vi "sweep(SubVI).vi"(0 "data":refnum<queue>, 1 "类型":enum16{"temp", "field", "position"}(ring), 2 "Instrument Ref In":refnum<k24>, 4 "config":refnum<queue>, 5 "steps number":i32, 7 "ch str":string, 9 "Field":dbl=300.0, 11 "Mode":i32(ring) items=["Persistent", "Driven"], 13 "Field 2":dbl=300.0, 14 "Rate、speed":dbl=10.0) -> (8 "错误输出":errorcluster)   [LabVIEW 2019, in "SubVI.lvlib"]
uses:
  SubVI.lvlib
  lib/QDInstrument.dll
  config.ctl
panel:
  out "Field\nStatus 3":i32(ring) items=["MagnetUnknown"=0, "StablePersistent"=1, "WarmingSwitch"=2, "CoolingSwitch"=3, "StableDriven"=4, "Iterating"=5, "Charging"=6, "Discharging"=7, "CurrentError"=8, "MagnetFailure"=15]
  out "Temperature\nStatus 2":i32(ring) items=["TemperatureUnknown"=0, "Stable"=1, "Tracking"=2, "Near"=5, "Chasing"=6, "Filling"=7, "Standby"=10, "Disabled"=13, "ImpedanceNotFunction"=14, "TempFailure"=15]
  out "Temperature\nStatus":i32(ring) items=["TemperatureUnknown"=0, "Stable"=1, "Tracking"=2, "Near"=5, "Chasing"=6, "Filling"=7, "Standby"=10, "Disabled"=13, "ImpedanceNotFunction"=14, "TempFailure"=15]
  out "Field\nStatus 2":i32(ring) items=["MagnetUnknown"=0, "StablePersistent"=1, "WarmingSwitch"=2, "CoolingSwitch"=3, "StableDriven"=4, "Iterating"=5, "Charging"=6, "Discharging"=7, "CurrentError"=8, "MagnetFailure"=15]
  # "(真是通道1，假是通道2)"
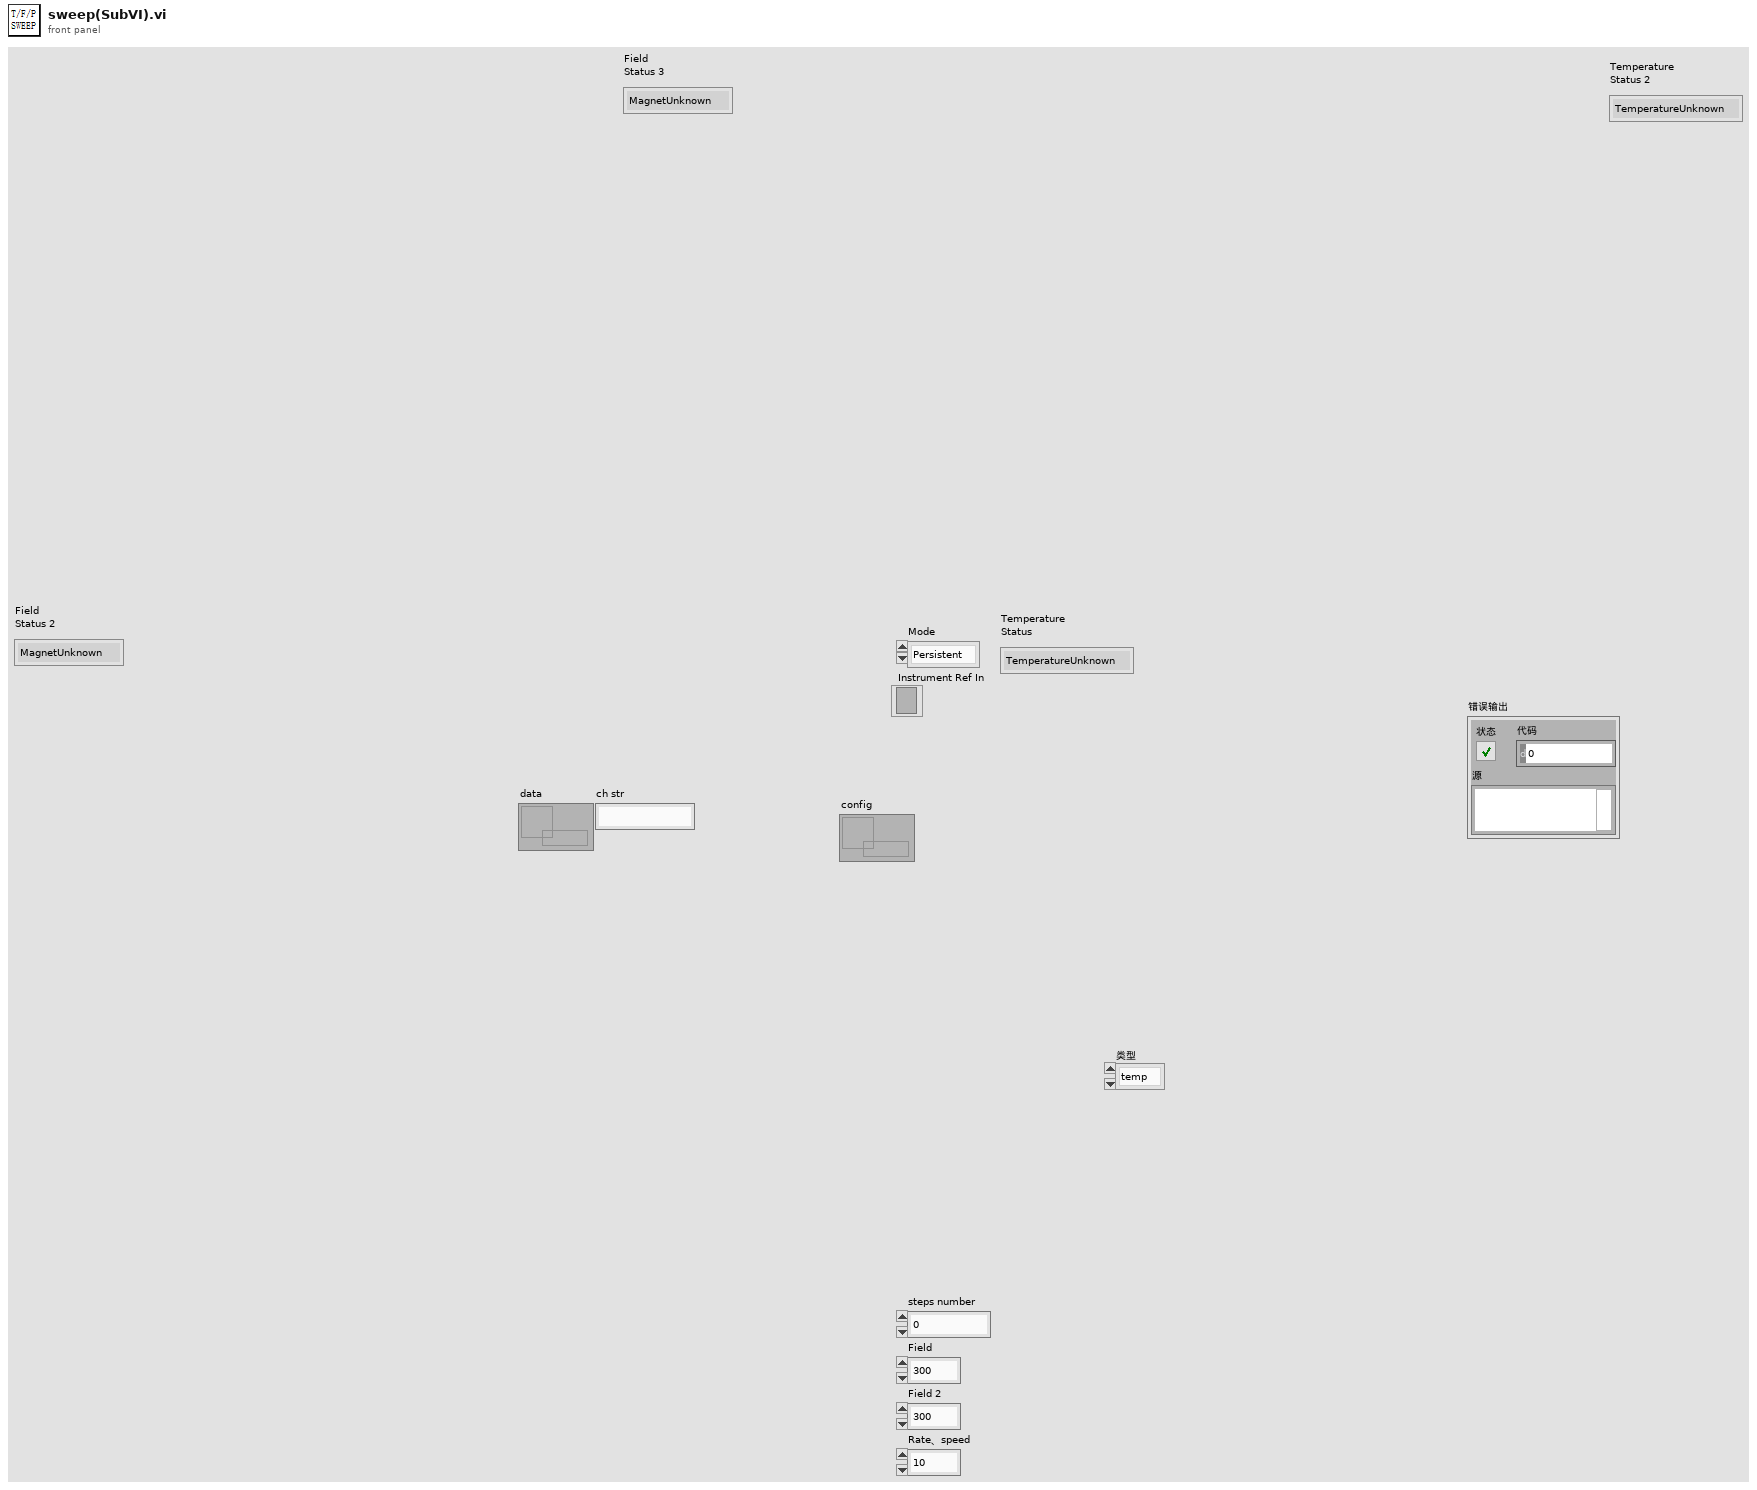
[diagram p1: front panel]
types:
  T1 = typedef "config.ctl" = cluster{"error":bool, "initialize":string, "数值":dbl, "6221":cluster{"6221 Resource":refnum<visa-resource-name>, "Delta status":bool}, "7001":cluster{"Ch":bool}}
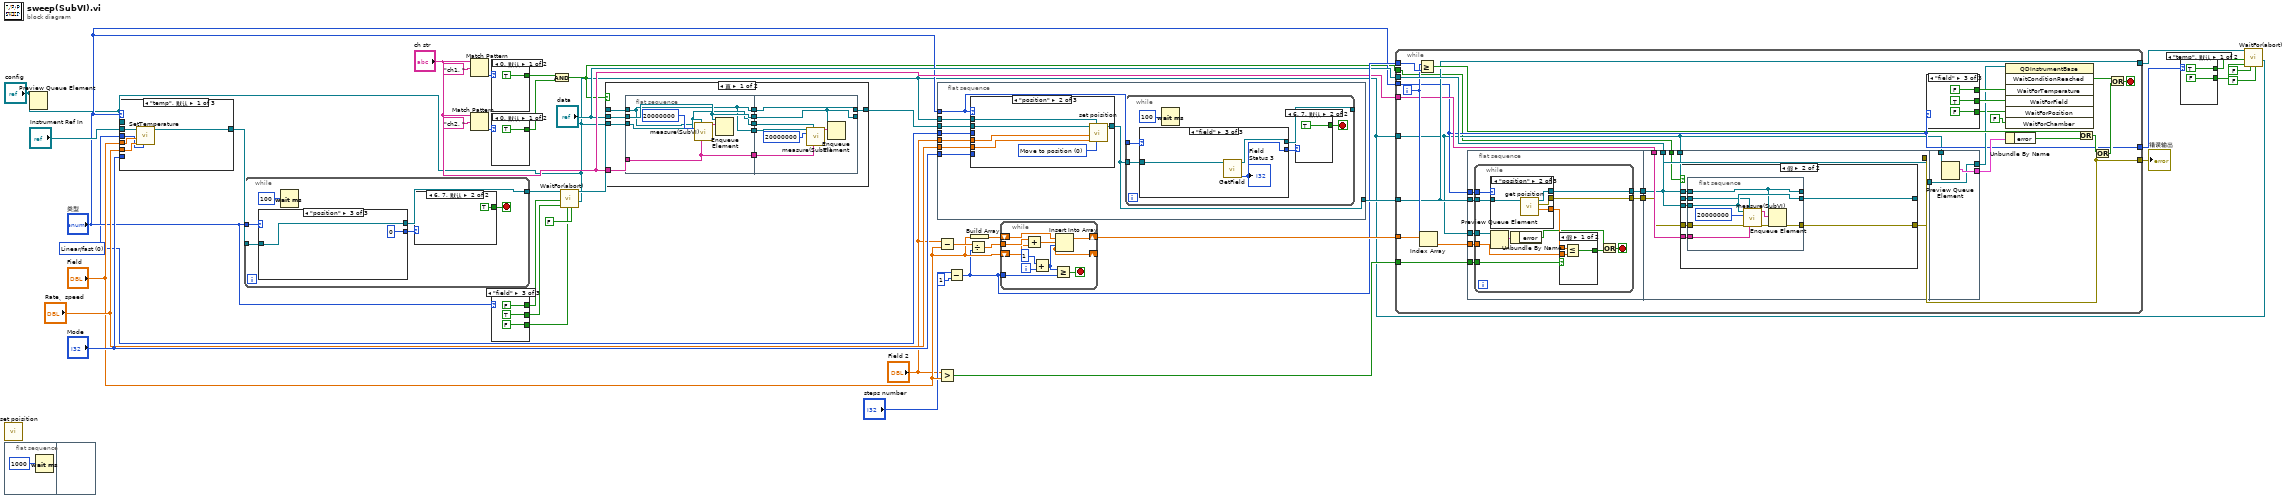
[diagram p0: block diagram]
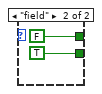
[diagram p2: hidden frame]
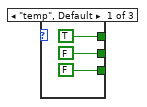
[diagram p3: hidden frame]
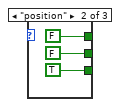
[diagram p4: hidden frame]
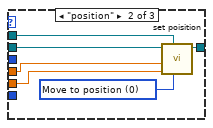
[diagram p5: hidden frame]
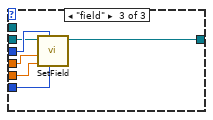
[diagram p6: hidden frame]
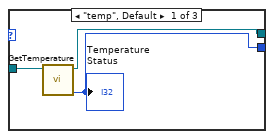
[diagram p7: hidden frame]
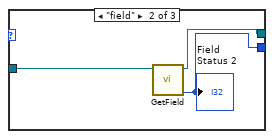
[diagram p8: hidden frame]
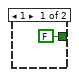
[diagram p9: hidden frame]
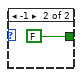
[diagram p10: hidden frame]
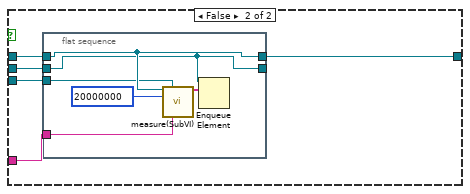
[diagram p11: hidden frame]
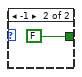
[diagram p12: hidden frame]
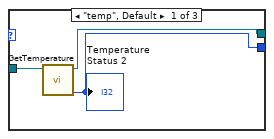
[diagram p13: hidden frame]
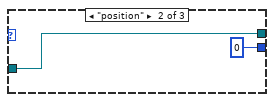
[diagram p14: hidden frame]
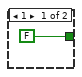
[diagram p15: hidden frame]
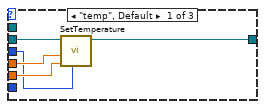
[diagram p16: hidden frame]
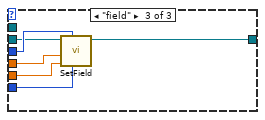
[diagram p17: hidden frame]
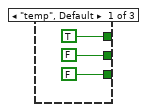
[diagram p18: hidden frame]
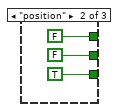
[diagram p19: hidden frame]
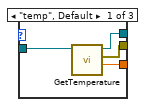
[diagram p20: hidden frame]
diagram:
  w5 = 0 items=["Linear/fast", "NoOvershoot", "Oscillate"] ("Approach")
  n1 = call "set poisition.vi"() -> ()  [unwired: 8 in, 2 out]
  n2 = flat-sequence {
    frame #0 {
      n3 = Wait (ms)(milliseconds to wait=u32 1000) -> ()  [unwired: 1 out]
    }
    frame #1 {
    }
  }
  n4 = Preview Queue Element(queue="config") -> ()  [unwired: 2 in, 4 out]
  n5 = case shown="\"temp\", 默认" "类型" {
    tunnel: "Rate、speed" -> [w45 w50 w59]
    tunnel: w5 -> [w43 _ w58]
    tunnel: "Mode" -> [_ _ w57]
    tunnel: "Instrument Ref In" -> [w47 w53 w56]
    tunnel: "Field" -> [w46 w51 w55]
    tunnel: [w44 w48 w54] -> w9
    tunnel: "config" -> [_ w49 _]
    frame "temp", Default {
      n6 = call "SetTemperature.vi"("Approach"=w43, "Rate"=w45, "Temperature"=w46, "Instrument Ref In"=w47) -> ("Instrument Ref Out"=w44:refnum<k24>)  [unwired: 3 in, 2 out]
    }
    frame "position" {
      w52 = u16 0 items=["Move to position", "Move to limit", "Redefine current position"] ("Mode")
      n7 = call "set poisition.vi"("Mode"=w52, "config"=w49, "Slow down code\ndefault = 0"=w50, "Position (deg)"=w51, "Instrument Ref In"=w53) -> ("Instrument Ref Out"=w48:refnum<k24>)  [unwired: 3 in, 1 out]
    }
    frame "field" {
      n8 = call "SetField.vi"("Mode"=w57, "Approach"=w58, "Rate"=w59, "Field"=w55, "Instrument Ref In"=w56) -> ("Instrument Ref Out"=w54:refnum<k24>)  [unwired: 2 in, 2 out]
    }
  }
  n9 = while {
    tunnel: w9 -> [w65]
    tunnel: [w61] -> w8
    tunnel: "类型" -> [w60]
    stop <- w63 stop-if-true
    n10 = case shown="\"position\"" w60 {
      tunnel: w65 -> [w68 w71 w73]
      tunnel: [w66 w70 0 ("Field\nStatus")] -> w64
      tunnel: [w67 w69 w73] -> w61
      frame "temp", Default {
        n11 = call "GetTemperature.vi"("Instrument Ref In"=w68) -> ("Temperature\nStatus"=w66:i32, "Instrument Ref Out"=w67:refnum<k24>)  [unwired: 4 in, 3 out]
        "Temperature\nStatus" <- w66
      }
      frame "field" {
        n12 = call "GetField.vi"("Instrument Ref In"=w71) -> ("Field\nStatus"=w70:i32, "Instrument Ref Out"=w69:refnum<k24>)  [unwired: 4 in, 3 out]
        "Field\nStatus 2" <- w70
      }
      frame "position" {
      }
    }
    n13 = Wait (ms)(milliseconds to wait=u32 100) -> ()  [unwired: 1 out]
    n14 = case shown="6, 7, 默认" w64 {
      tunnel: [FALSE TRUE] -> w63
      frame 1 {
      }
      frame 6, 7, Default {
      }
    }
  }
  n15 = Match Pattern(string="ch str", regular expression="ch1, " ("正则表达式")) -> (offset past match=w17:i32)  [unwired: 1 in, 3 out]
  n16 = Match Pattern(string="ch str", regular expression="ch2, " ("正则表达式")) -> (offset past match=w16:i32)  [unwired: 1 in, 3 out]
  n17 = case shown="0, 默认" w17 {
    tunnel: [TRUE FALSE] -> w15
    frame 0, Default {
    }
    frame -1 {
    }
  }
  n18 = case shown="0, 默认" w16 {
    tunnel: [TRUE FALSE] -> w14
    frame 0, Default {
    }
    frame -1 {
    }
  }
  n19 = case shown="\"field\"" "类型" {
    tunnel: [FALSE ("Wait For Field") FALSE ("Wait For Field") TRUE ("Wait For Field")] -> w21
    tunnel: [TRUE ("Wait For Temperature") FALSE ("Wait For Temperature") FALSE ("Wait For Temperature")] -> w20
    tunnel: [FALSE ("Wait For Position") TRUE ("Wait For Position") FALSE ("Wait For Position")] -> w4
    frame "temp", Default {
    }
    frame "position" {
    }
    frame "field" {
    }
  }
  n20 = And(x=w15, y=w14) -> (x .and. y?=w1:bool)
  n21 = call "WaitFor(abort).vi"("config"="config", "Wait For Chamber"=FALSE, "Wait For Position"=w4, "Wait For Field"=w21, "Wait For Temperature"=w20, "Instrument Ref In"=w8) -> ("Instrument Ref Out"=w13:refnum<k24>)  [unwired: 4 in, 1 out]
  n22 = case shown="真" w1 {
    tunnel: w13 -> [w98 w116]
    tunnel: "ch str" -> [w97 w115]
    tunnel: "data" -> [w96 w114]
    tunnel: "config" -> [w95 w113]
    tunnel: [w94 w112] -> w10
    frame True {
      n23 = flat-sequence {
        tunnel: w98 -> [w99]
        tunnel: w97 -> [w100]
        tunnel: w96 -> [w102]
        tunnel: w95 -> [w101]
        tunnel: [w99] -> w93
        tunnel: [w102] -> w92
        tunnel: [w101] -> w91
        tunnel: [w100] -> w90
        tunnel: [w99] -> w89
        tunnel: [w105] -> _
        tunnel: [w111] -> w94
        tunnel: w93 -> [w111]
        tunnel: w92 -> [w105]
        tunnel: w91 -> [w108]
        tunnel: w90 -> [w107]
        tunnel: w89 -> [w106]
        frame #0 {
          n24 = call "measure(SubVI).vi"(".NET引用句柄输入"=w99, "config"=w101, "Timeout (20000 ms)"=u32 20000000, "ch str"=w100) -> ("data"=w103:string[])  [unwired: 10 in, 1 out]
          n25 = Enqueue Element(queue=w102, element=w103) -> ()  [unwired: 2 in, 3 out]
        }
        frame #1 {
          n26 = call "measure(SubVI).vi"(".NET引用句柄输入"=w106, "config"=w108, "Timeout (20000 ms)"=u32 20000000, "ch str"=w107) -> ("data"=w110:string[])  [unwired: 10 in, 1 out]
          n27 = Enqueue Element(queue=w105, element=w110) -> ()  [unwired: 2 in, 3 out]
        }
      }
    }
    frame False {
      n28 = flat-sequence {
        tunnel: w116 -> [w122]
        tunnel: [w122] -> w112
        tunnel: w115 -> [w120]
        tunnel: [w118] -> _
        tunnel: w114 -> [w118]
        tunnel: w113 -> [w117]
        frame #0 {
          n29 = call "measure(SubVI).vi"(".NET引用句柄输入"=w122, "config"=w117, "Timeout (20000 ms)"=u32 20000000, "ch str"=w120) -> ("data"=w119:string[])  [unwired: 10 in, 1 out]
          n30 = Enqueue Element(queue=w118, element=w119) -> ()  [unwired: 2 in, 3 out]
        }
      }
    }
  }
  n31 = flat-sequence {
    tunnel: "Field 2" -> [w127]
    tunnel: "Rate、speed" -> [w128]
    tunnel: w5 -> [w130]
    tunnel: "Mode" -> [w126]
    tunnel: [w125] -> w32
    tunnel: w10 -> [w129]
    tunnel: "类型" -> [w124]
    tunnel: "config" -> [w123]
    frame #0 {
      n32 = case shown="\"position\"" w124 {
        tunnel: w128 -> [w149 w154 w163]
        tunnel: w130 -> [w147 _ w162]
        tunnel: w126 -> [_ _ w161]
        tunnel: w129 -> [w151 w156 w160]
        tunnel: w127 -> [w150 w155 w159]
        tunnel: [w148 w157 w158] -> w125
        tunnel: w123 -> [_ w152 _]
        frame "temp", Default {
          n33 = call "SetTemperature.vi"("Approach"=w147, "Rate"=w149, "Temperature"=w150, "Instrument Ref In"=w151) -> ("Instrument Ref Out"=w148:refnum<k24>)  [unwired: 3 in, 2 out]
        }
        frame "position" {
          w153 = u16 0 items=["Move to position", "Move to limit", "Redefine current position"] ("Mode")
          n34 = call "set poisition.vi"("Mode"=w153, "config"=w152, "Slow down code\ndefault = 0"=w154, "Position (deg)"=w155, "Instrument Ref In"=w156) -> ("Instrument Ref Out"=w157:refnum<k24>)  [unwired: 3 in, 1 out]
        }
        frame "field" {
          n35 = call "SetField.vi"("Mode"=w161, "Approach"=w162, "Rate"=w163, "Field"=w159, "Instrument Ref In"=w160) -> ("Instrument Ref Out"=w158:refnum<k24>)  [unwired: 2 in, 2 out]
        }
      }
      n36 = while {
        tunnel: w125 -> [w136]
        tunnel: [w132] -> _
        tunnel: w124 -> [w131]
        stop <- w134 stop-if-true
        n37 = case shown="\"field\"" w131 {
          tunnel: w136 -> [w139 w140 w144]
          tunnel: [w137 0 ("Field\nStatus") w143] -> w135
          tunnel: [w138 w140 w142] -> w132
          frame "temp", Default {
            n38 = call "GetTemperature.vi"("Instrument Ref In"=w139) -> ("Temperature\nStatus"=w137:i32, "Instrument Ref Out"=w138:refnum<k24>)  [unwired: 4 in, 3 out]
            "Temperature\nStatus 2" <- w137
          }
          frame "position" {
          }
          frame "field" {
            n39 = call "GetField.vi"("Instrument Ref In"=w144) -> ("Field\nStatus"=w143:i32, "Instrument Ref Out"=w142:refnum<k24>)  [unwired: 4 in, 3 out]
            "Field\nStatus 3" <- w143
          }
        }
        n40 = Wait (ms)(milliseconds to wait=u32 100) -> ()  [unwired: 1 out]
        n41 = case shown="6, 7, 默认" w135 {
          tunnel: [FALSE TRUE] -> w134
          frame 1 {
          }
          frame 6, 7, Default {
          }
        }
      }
    }
  }
  n42 = Subtract(x="Field 2", y="Field") -> (x-y=w41:dbl)
  n43 = Greater?(x="Field 2", y="Field") -> (0:w34:bool)
  n44 = Subtract(x="steps number", y=1) -> (x-y=w23:i32)
  n45 = Divide(x=w41, y=w23) -> (x/y=w39:dbl)
  n46 = Build Array("Field") -> (w40:dbl[])
  n47 = while {
    shift-right: [w173] -> w36
    shift-left: w40 -> [w172]
    tunnel: w39 -> [w167]
    tunnel: w23 -> [w166]
    shift-right: [w165] -> _
    shift-left: "Field" -> [w164]
    i -> [w171]
    stop <- w168 stop-if-true
    n48 = Add(x=w167, y=w164) -> (x+y=w165:dbl)
    n49 = Add(x=1, y=w171) -> (x+y=w169:i32)
    n50 = Greater Or Equal?(x=w169, y=w166) -> (x >= y?=w168:bool)
    n51 = Insert Into Array(array=w172, index=w169, new element=w165) -> (w173:dbl[])
  }
  n52 = while {
    tunnel: w36 -> [w200]
    tunnel: w23 -> [w196]
    tunnel: "data" -> [w198]
    tunnel: "config" -> [w176]
    tunnel: w32 -> [w192]
    tunnel: w34 -> [w194]
    tunnel: [w192] -> w27
    tunnel: [w190] -> w26
    tunnel: "ch str" -> [w180]
    tunnel: "类型" -> [w177]
    tunnel: [w177] -> w6
    tunnel: w1 -> [w174]
    i -> [w195]
    stop <- w181 stop-if-true
    n53 = Greater Or Equal?(x=w195, y=w196) -> (x >= y?=w197:bool)
    n54 = Index Array(array=w200, index=w195) -> (element=w193:dbl)
    n55 = flat-sequence {
      tunnel: [w213] -> w199
      tunnel: w192 -> [w216]
      tunnel: w194 -> [w215]
      tunnel: w193 -> [w214]
      tunnel: w176 -> [w212]
      tunnel: [w211] -> w191
      tunnel: w177 -> [w210]
      tunnel: w199 -> [w252]
      tunnel: w198 -> [w250]
      tunnel: w176 -> [w251]
      tunnel: w191 -> [w247]
      tunnel: [w248] -> w190
      tunnel: [w252] -> w184
      tunnel: w180 -> [w253]
      tunnel: w174 -> [w249]
      tunnel: w176 -> [w304]
      tunnel: [w303] -> w179
      tunnel: [w302] -> w185
      tunnel: w184 -> [w302]
      frame #0 {
        n56 = while {
          tunnel: w216 -> [w226]
          tunnel: w215 -> [w228]
          tunnel: w214 -> [w227]
          tunnel: [w220] -> w213
          tunnel: w212 -> [w224]
          tunnel: [w221] -> w211
          tunnel: w210 -> [w217]
          stop <- w222 stop-if-true
          n57 = case shown="\"position\"" w217 {
            tunnel: w226 -> [w229 w236 w240]
            tunnel: [w230 w233 w239] -> w225
            tunnel: [w231 w234 w238] -> w221
            tunnel: [w232 w235 w237] -> w220
            frame "temp", Default {
              n58 = call "GetTemperature.vi"("Instrument Ref In"=w229) -> ("Temperature"=w230:dbl, "error out"=w231:errorcluster, "Instrument Ref Out"=w232:refnum<k24>)  [unwired: 4 in, 2 out]
            }
            frame "position" {
              n59 = call "get poisition.vi"("Instrument Ref In"=w236) -> ("Position"=w233:dbl, "error out"=w234:errorcluster, "Instrument Ref Out 2"=w235:refnum<k24>)  [unwired: 4 in]
            }
            frame "field" {
              n60 = call "GetField.vi"("Instrument Ref In"=w240) -> ("Field"=w239:dbl, "error out"=w238:errorcluster, "Instrument Ref Out"=w237:refnum<k24>)  [unwired: 4 in, 2 out]
            }
          }
          n61 = Preview Queue Element(queue=w224) -> (element=w219:T1)  [unwired: 2 in, 3 out]
          n62 = Unbundle By Name(w219) -> ("error"=w218:bool)
          n63 = case shown="假" w228 {
            tunnel: w225 -> [w243 w246]
            tunnel: w227 -> [w242 w245]
            tunnel: [w241 w244] -> w223
            frame False {
              n64 = Less Or Equal?(x=w243, y=w242) -> (x <= y?=w241:bool)
            }
            frame True {
              n65 = Greater Or Equal?(x=w246, y=w245) -> (x >= y?=w244:bool)
            }
          }
          n66 = Or(x=w218, y=w223) -> (x .or. y?=w222:bool)
        }
      }
      frame #1 {
        n67 = case shown="假" w249 {
          tunnel: w252 -> [w266 w292]
          tunnel: w253 -> [w265 w291]
          tunnel: w250 -> [w264 w290]
          tunnel: w251 -> [w263 w289]
          tunnel: [w262 w288] -> _
          tunnel: [w256 w287] -> w248
          tunnel: w247 -> [w254 w286]
          frame True {
            n68 = flat-sequence {
              tunnel: w266 -> [w270]
              tunnel: w265 -> [w271]
              tunnel: w264 -> [w273]
              tunnel: w263 -> [w272]
              tunnel: [w270] -> w261
              tunnel: [w273] -> w260
              tunnel: [w272] -> w259
              tunnel: [w271] -> w258
              tunnel: [w270] -> w257
              tunnel: [w269] -> w255
              tunnel: w254 -> [w267]
              tunnel: [w279] -> _
              tunnel: [w285] -> w262
              tunnel: w261 -> [w285]
              tunnel: w260 -> [w279]
              tunnel: w259 -> [w282]
              tunnel: w258 -> [w281]
              tunnel: w257 -> [w280]
              tunnel: [w278] -> w256
              tunnel: w255 -> [w276]
              frame #0 {
                n69 = call "measure(SubVI).vi"(".NET引用句柄输入"=w270, "config"=w272, "Timeout (20000 ms)"=u32 20000000, "error in (no error)"=w267, "ch str"=w271) -> ("data"=w274:string[], "error out"=w268:errorcluster)  [unwired: 9 in]
                n70 = Enqueue Element(queue=w273, element=w274, error in (no error)=w268) -> (error out=w269:errorcluster)  [unwired: 1 in, 2 out]
              }
              frame #1 {
                n71 = call "measure(SubVI).vi"(".NET引用句柄输入"=w280, "config"=w282, "Timeout (20000 ms)"=u32 20000000, "error in (no error)"=w276, "ch str"=w281) -> ("data"=w284:string[], "error out"=w277:errorcluster)  [unwired: 9 in]
                n72 = Enqueue Element(queue=w279, element=w284, error in (no error)=w277) -> (error out=w278:errorcluster)  [unwired: 1 in, 2 out]
              }
            }
          }
          frame False {
            n73 = flat-sequence {
              tunnel: w292 -> [w301]
              tunnel: [w301] -> w288
              tunnel: w291 -> [w299]
              tunnel: [w297] -> _
              tunnel: w290 -> [w297]
              tunnel: w289 -> [w296]
              tunnel: [w295] -> w287
              tunnel: w286 -> [w293]
              frame #0 {
                n74 = call "measure(SubVI).vi"(".NET引用句柄输入"=w301, "config"=w296, "Timeout (20000 ms)"=u32 20000000, "error in (no error)"=w293, "ch str"=w299) -> ("data"=w298:string[], "error out"=w294:errorcluster)  [unwired: 9 in]
                n75 = Enqueue Element(queue=w297, element=w298, error in (no error)=w294) -> (error out=w295:errorcluster)  [unwired: 1 in, 2 out]
              }
            }
          }
        }
      }
      frame #2 {
        n76 = Preview Queue Element(queue=w304) -> (element=w303:T1)  [unwired: 2 in, 3 out]
      }
    }
    n77 = case shown="\"field\"" w177 {
      tunnel: [FALSE ("WaitForField") FALSE ("WaitForField") TRUE ("WaitForField")] -> w188
      tunnel: [TRUE ("WaitForTemperature") FALSE ("WaitForTemperature") FALSE ("WaitForTemperature")] -> w186
      tunnel: [FALSE ("WaitForPosition") TRUE ("WaitForPosition") FALSE ("WaitForPosition")] -> w175
      frame "temp", Default {
      }
      frame "position" {
      }
      frame "field" {
      }
    }
    n78 = Unbundle By Name(w179) -> ("error"=w178:bool)
    n79 = invoke class="QDInstrumentBase" method="WaitConditionReached"(reference=w185, "WaitForTemperature"=w186, "WaitForField"=w188, "WaitForPosition"=w175, "WaitForChamber"=FALSE) -> ("WaitConditionReached"=w183:bool)  [unwired: 2 in, 6 out]
    n80 = Or(x=w197, y=w178) -> (x .or. y?=w189:bool)
    n81 = Or(x=w189, y=w190) -> (x .or. y?=w182:bool)
    n82 = Or(x=w183, y=w182) -> (x .or. y?=w181:bool)
  }
  "错误输出" <- w26
  n83 = case shown="\"temp\", 默认" w6 {
    tunnel: [FALSE ("Wait For Field") TRUE ("Wait For Field")] -> w29
    tunnel: [TRUE ("Wait For Temperature") FALSE ("Wait For Temperature")] -> w28
    frame "temp", Default {
    }
    frame "field" {
    }
  }
  n84 = call "WaitFor(abort).vi"("config"="config", "Wait For Chamber"=FALSE, "Wait For Position"=FALSE, "Wait For Field"=w29, "Wait For Temperature"=w28, "Instrument Ref In"=w27) -> ()  [unwired: 4 in, 2 out]
